vi "GetTeleopAuto.vi"(11 "DriveBase in":refnum<class "DriveBase.lvclass">) -> (2 "Teleop or Auto":enum16{"Teleop", "Autonomous"}(ring), 3 "DriveBase out":refnum<class "DriveBase.lvclass">)   [LabVIEW 2016]
uses:
  DriveBase.lvclass
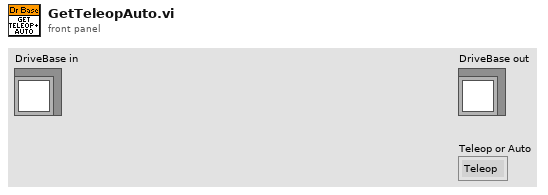
[diagram p1: front panel]
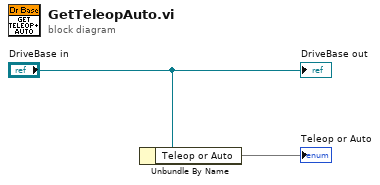
[diagram p0: block diagram]
diagram:
  n1 = Unbundle By Name("DriveBase in") -> ("Teleop or Auto"=→"Teleop or Auto")
  "DriveBase out" <- "DriveBase in"
